vi "Write Waveform.vi"(8 "error in (no error)":errorcluster, 10 "I-V parameters":T1={"Start magnitude"=0.001, "Magnitude increment"=0.001, "End magnitude"=0.01, "Ramp length"=0, "Top  length"=0, "Threshold "=2e-06, "Processing delay"=0, "Valhalla range"=0.001, "Interpolation"=64, "Stop after"=1, "Detector window"=480} {"Detector window" format="%dpts"; "Stop after" format="%d sweep(s)"; "Valhalla range" format="%#_6pA"; "Processing delay" format="%dpts"; "Threshold" format="%#_6pV"; "Top  length" format="%dpts"; "Ramp length" format="%dpts"; "End magnitude" format="%#_6pA"; "Magnitude increment" format="%#_6pA"; "Start magnitude" format="%#_6pA"}, 11 "RP Instrument in":refnum<class "RP Instrument.lvclass">) -> (0 "error out":errorcluster, 2 "Output Waveform":i16[](graph), 3 "RP Instrument out":refnum<class "RP Instrument.lvclass">)   [LabVIEW 2016, in "RP Instrument.lvclass"]
uses:
  RP Instrument.lvclass
  Waform generation/I-V parameters.ctl
  RP Instrument.lvclass/RP Instrument.ctl
  RP Communicator/RP Communicator.lvclass
panel:
  # "Waveform parameters"
  # "Detector parameters"
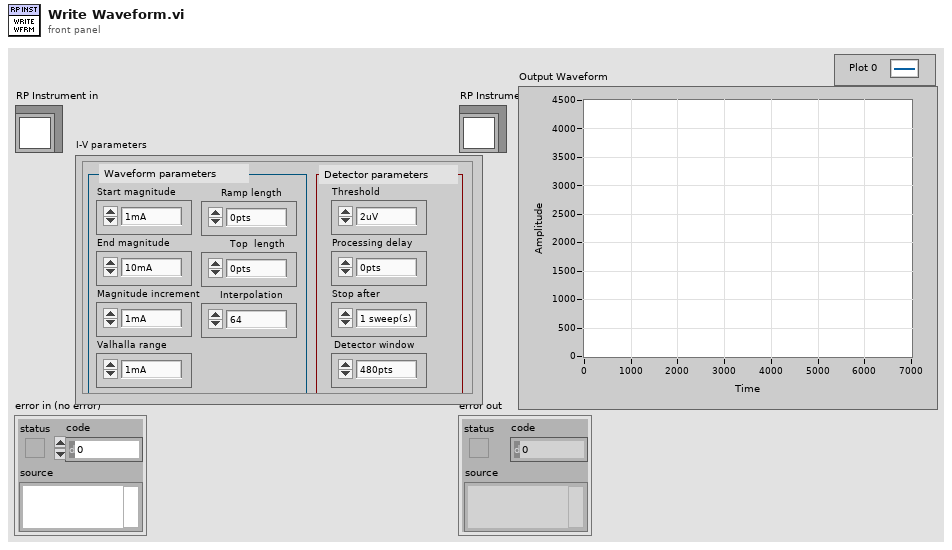
[diagram p1: front panel]
types:
  T1 = typedef "I-V parameters.ctl" = cluster{"Start magnitude":dbl, "Magnitude increment":dbl, "End magnitude":dbl, "Ramp length":i32, "Top  length":i32, "Threshold ":dbl, "Processing delay":u16, "Valhalla range":dbl, "Interpolation":i32, "Stop after":u16, "Detector window":i32}
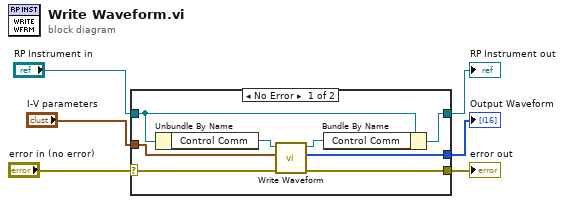
[diagram p0: block diagram]
diagram:
  n1 = case shown="No Error" "error in (no error)" {
    selector: "error in (no error)" -> [w9 w16]
    tunnel: [w8 w16] -> w5
    tunnel: [w12 w15] -> w3
    tunnel: "RP Instrument in" -> [w14 w15]
    tunnel: "I-V parameters" -> [w10 _]
    tunnel: [w7 _] -> w1
    frame No Error {
      n2 = Unbundle By Name(w14) -> ("Control Comm"=w13:refnum<class "RP Communicator.lvclass">)
      n3 = call-dynamic "Write Waveform.vi"("error in (no error)"=w9, "I-V parameters"=w10, "RP Communicator in"=w13) -> ("error out"=w8:errorcluster, "Output Waveform"=w7:i16[], "RP Communicator out"=w11:refnum<class "RP Communicator.lvclass">)  [unwired: 6 in]
      n4 = Bundle By Name(cluster=w14, "Control Comm"=w11) -> (w12:refnum<class "RP Instrument.lvclass">)
    }
    frame Error {
    }
  }
  "error out" <- w5
  "RP Instrument out" <- w3
  "Output Waveform" <- w1
